vi "Inst_CNT90.vi"(8 "error in":errorcluster, 10 "All Message Queues in":T1, 11 "AjustesPrevios in":refnum<class "AjustesPrevios.lvclass">) -> (0 "error out":errorcluster)   [LabVIEW 2019, in "AjustesPrevios.lvclass"]
uses:
  AjustesPrevios.lvclass
  QMH/Message Queue/All Message Queues.ctl
  QMH/Message Queue/Message Cluster.ctl
  AjustesPrevios.lvclass/AjustesPrevios.ctl
  <vilib>/Utility/error.llb/Error Cluster From Error Code.vi
  QMH/Message Queue/Enqueue Message (Single).vi
  <vilib>/ErrorRing/Error Ring.xnode
  QMH/Message Queue/Message Queue.lvlib
  Instrumento/CNT90/CNT90.lvclass
panel:
  out "All States":string[](array[string])
  out "Actual State":string
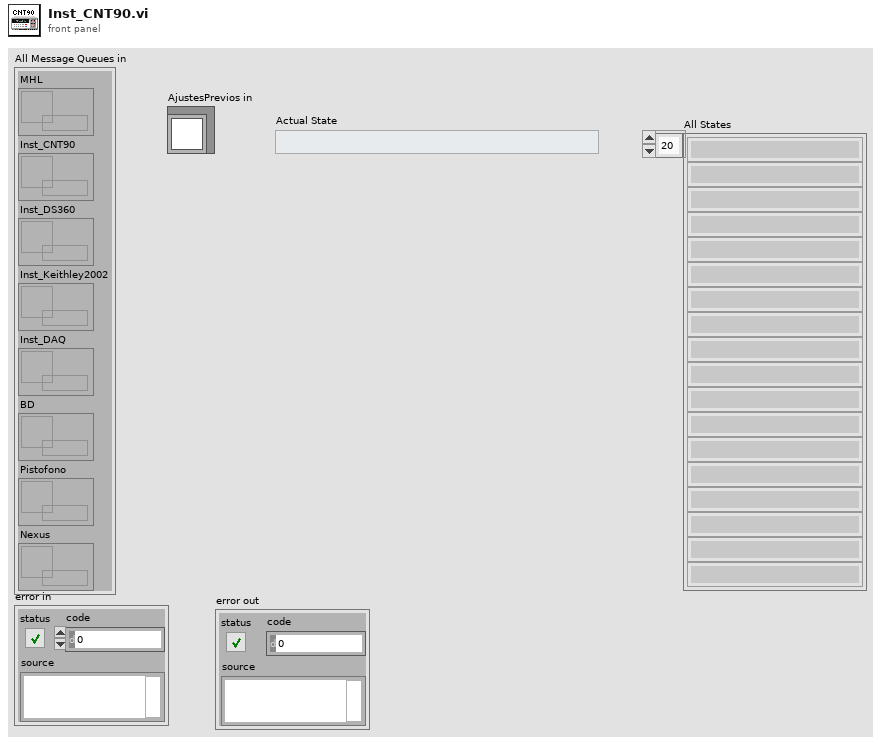
[diagram p1: front panel]
types:
  T1 = typedef "Message Queue.lvlib/All Message Queues.ctl" = cluster{"MHL":refnum<queue>, "Inst_CNT90":refnum<queue>, "Inst_DS360":refnum<queue>, "Inst_Keithley2002":refnum<queue>, "Inst_DAQ":refnum<queue>, "BD":refnum<queue>, "Pistofono":refnum<queue>, "Nexus":refnum<queue>}
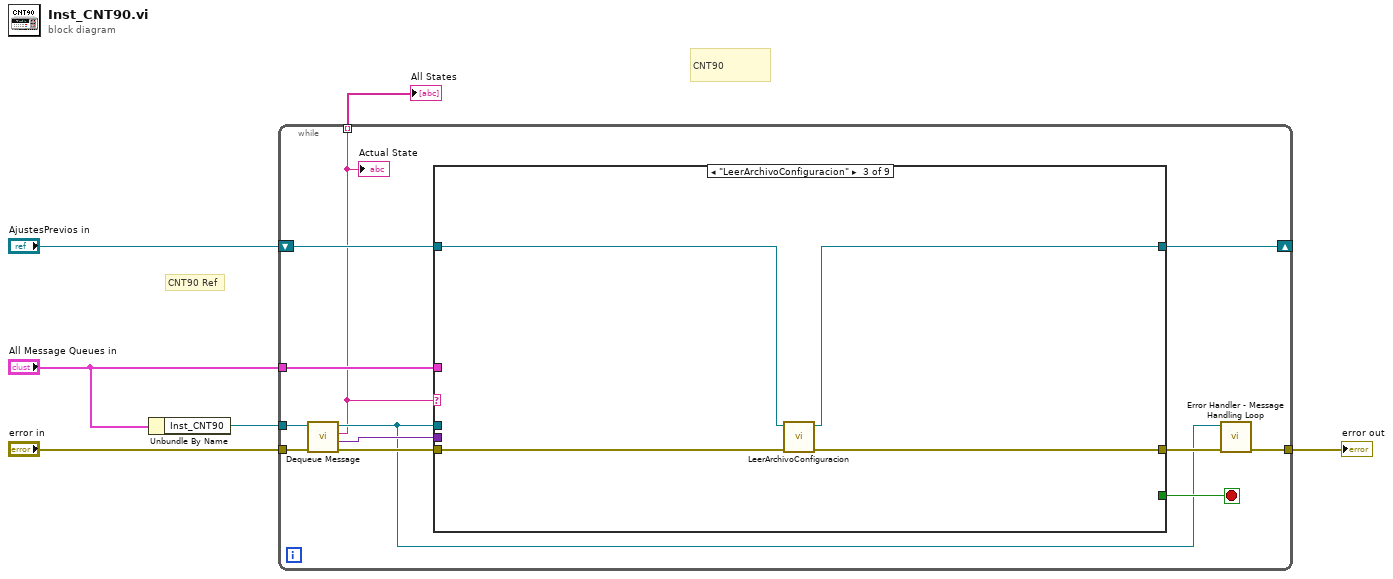
[diagram p0: block diagram]
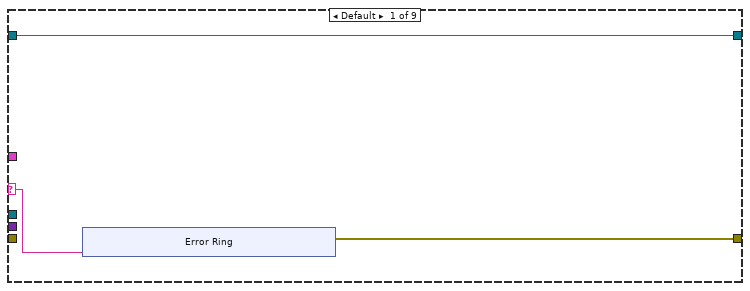
[diagram p2: hidden frame]
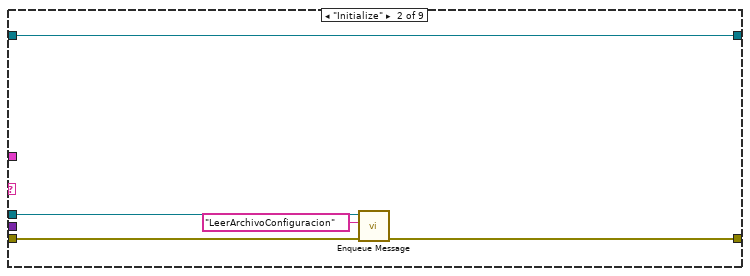
[diagram p3: hidden frame]
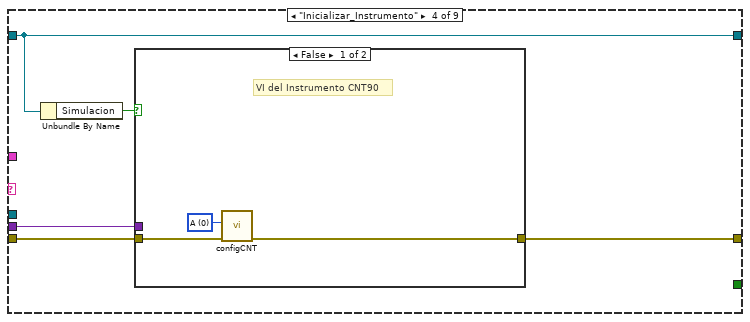
[diagram p4: hidden frame]
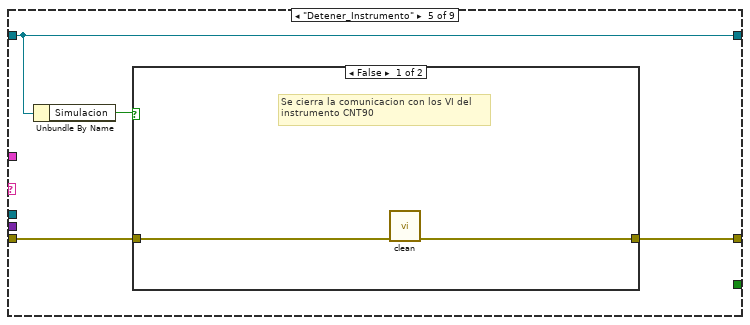
[diagram p6: hidden frame]
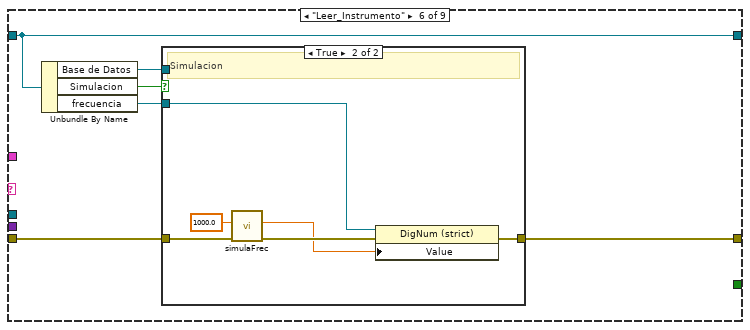
[diagram p8: hidden frame]
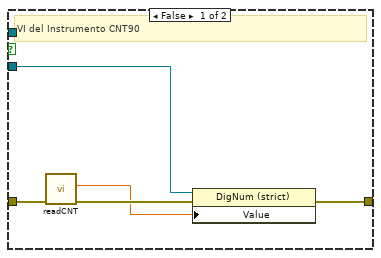
[diagram p9: hidden frame]
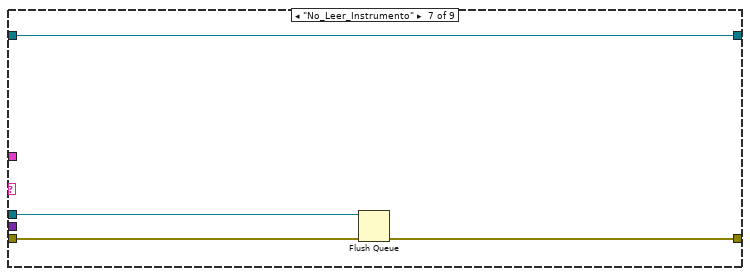
[diagram p10: hidden frame]
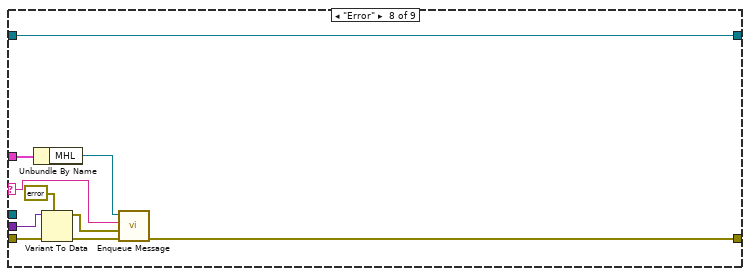
[diagram p11: hidden frame]
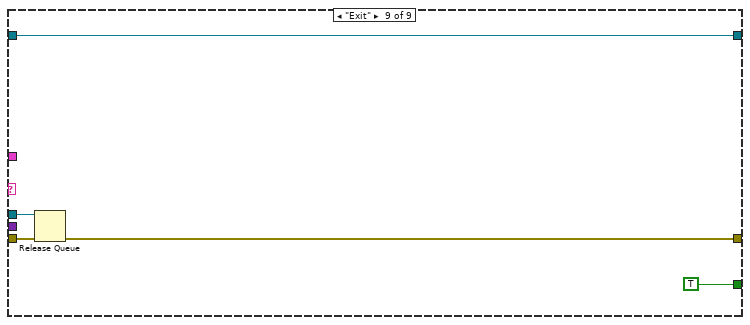
[diagram p12: hidden frame]
diagram:
  # "CNT90"
  # "CNT90 Ref"
  n1 = Unbundle By Name("All Message Queues in") -> ("Inst_CNT90"=w5:refnum<queue>)
  n2 = while {
    tunnel: "error in" -> [w18]
    tunnel: w5 -> [w17]
    tunnel: "All Message Queues in" -> [w16]
    tunnel: [w9] -> w3
    shift-right: [w12] -> _
    shift-left: "AjustesPrevios in" -> [w15]
    tunnel: [w7] -> w2 mode=indexing
    stop <- w11 stop-if-true
    n3 = call "Dequeue Message.vi"("error in (no error)"=w18, "Message Queue"=w17) -> ("error out"=w13:errorcluster, "Message Data"=w14:variant, "Message"=w7:string, "dup Message Queue"=w8:refnum<queue>)  [unwired: 6 in]
    "Actual State" <- w7
    n4 = case shown="\"LeerArchivoConfiguracion\"" w7 {
      selector: w7 -> [w21 _ _ _ _ _ _ w79 _]
      tunnel: w16 -> [_ _ _ _ _ _ _ w78 _]
      tunnel: w15 -> [w19 w33 w35 w42 w49 w57 w73 w76 w86]
      tunnel: w8 -> [_ w30 _ _ _ _ w71 _ w88]
      tunnel: w14 -> [_ _ _ w38 _ _ _ w82 _]
      tunnel: w13 -> [_ w32 w37 w41 w47 w59 w74 w83 w89]
      tunnel: [w20 w31 w36 w39 w50 w58 w72 w75 w85] -> w10
      tunnel: [w19 w33 w34 w42 w49 w57 w73 w76 w86] -> w12
      tunnel: [_ _ _ _ _ _ _ _ TRUE] -> w11
      frame Default {
        n5 = xnode "Error Ring"("parameter 0"=w21) -> ("error out"=w20:errorcluster)
      }
      frame "Initialize" {
        n6 = call-poly "Enqueue Message.vi"("error in (no error)"=w32, "Message"="LeerArchivoConfiguracion", "Message Queue"=w30) -> ("error out"=w31:errorcluster)  [unwired: 7 in, 1 out]
      }
      frame "LeerArchivoConfiguracion" {
        n7 = call "LeerArchivoConfiguracion.vi"("error in"=w37, "AjustesPrevios in"=w35) -> ("error out"=w36:errorcluster, "AjustesPrevios out"=w34:refnum<class "AjustesPrevios.lvclass">)  [unwired: 8 in]
      }
      frame "Inicializar_Instrumento" {
        n8 = Unbundle By Name(w42) -> ("Simulacion"=w40:bool)
        n9 = case shown="False" w40 {
          tunnel: [w45 w46] -> w39
          tunnel: w41 -> [w44 w46]
          tunnel: w38 -> [_ _]
          frame False {
            w43 = 0 items=["A", "B"] ("Channel  1")
            # "VI del Instrumento CNT90"
            n10 = call "configCNT.vi"("error in (no error)"=w44, "Channel  1"=w43) -> ("error out"=w45:errorcluster)  [unwired: 8 in, 1 out]
          }
          frame True {
            # "Simulacion"
          }
        }
      }
      frame "Detener_Instrumento" {
        n11 = Unbundle By Name(w49) -> ("Simulacion"=w48:bool)
        n12 = case shown="False" w48 {
          tunnel: [w52 w53] -> w50
          tunnel: w47 -> [w51 w53]
          frame False {
            # "Se cierra la comunicacion con los VI del\ninstrumento CNT90"
            n13 = call "clean.vi"("error in (no error)"=w51) -> ("error out"=w52:errorcluster)  [unwired: 9 in, 1 out]
          }
          frame True {
            # "Simulacion"
          }
        }
      }
      frame "Leer_Instrumento" {
        n14 = Unbundle By Name(w57) -> ("Base de Datos"=w55:refnum<class "Base de Datos.lvclass">, "Simulacion"=w56:bool, "frecuencia"=w54:refnum<vi>)
        n15 = case shown="True" w56 {
          tunnel: [w62 w67] -> w58
          tunnel: w59 -> [w64 w70]
          tunnel: w55 -> [_ _]
          tunnel: w54 -> [w61 w66]
          frame False {
            # "VI del Instrumento CNT90"
            n16 = call "readCNT.vi"("error in (no error)"=w64) -> ("error out"=w63:errorcluster, "medicion"=w60:dbl)  [unwired: 8 in, 1 out]
            n17 = property class="DigNum (strict)"(reference=w61, error in=w63, "Value"=w60) -> (error out=w62:errorcluster)  [unwired: 1 out]
          }
          frame True {
            # "Simulacion"
            n18 = call "simulaFrec.vi"("error in (no error)"=w70, "frec in"=1000.0) -> ("error out"=w68:errorcluster, "frec out"=w65:dbl)  [unwired: 7 in, 1 out]
            n19 = property class="DigNum (strict)"(reference=w66, error in=w68, "Value"=w65) -> (error out=w67:errorcluster)  [unwired: 1 out]
          }
        }
      }
      frame "No_Leer_Instrumento" {
        n20 = Flush Queue(queue=w71, error in (no error)=w74) -> (error out=w72:errorcluster)  [unwired: 2 out]
      }
      frame "Error" {
        n21 = Unbundle By Name(w78) -> ("MHL"=w77:refnum<queue>)
        n22 = Variant To Data(error in=w83, type=errorcluster {"status"=FALSE, "code"=0, "source"=""} ("error constant"), Variant=w82) -> (data=w80:errorcluster, error out=w81:errorcluster)
        n23 = call-poly "Enqueue Message.vi"("error in (no error)"=w81, "Message Data"=w80, "Message"=w79, "Message Queue"=w77) -> ("error out"=w75:errorcluster)  [unwired: 6 in, 1 out]
      }
      frame "Exit" {
        n24 = Release Queue(queue=w88, error in (no error)=w89) -> (error out=w85:errorcluster)  [unwired: 1 in, 2 out]
      }
    }
    n25 = call "Error Handler - Message Handling Loop.vi"("error in (no error)"=w10, "Message Queue"=w8) -> ("dup error in"=w9:errorcluster)  [unwired: 8 in, 1 out]
  }
  "error out" <- w3
  "All States" <- w2
